vi "Describe Variant.vi"(11 "Variant":variant) -> (1 "Type Description":string, 2 "Description":string, 3 "Variant Description":string)   [LabVIEW 2020, in "LUnit Test Case.lvclass"]
uses:
  LUnit Test Case.lvclass
  <vilib>/Utility/Data Type/NI_Data Type.lvlib
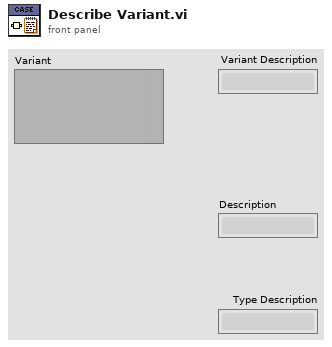
[diagram p1: front panel]
types:
  T1 = typedef "NI_Data Type.lvlib/Data Type.ctl" = enum8{"Invalid Type", "Void", "I8", "I16", "I32", "I64", "U8", "U16", "U32", "U64", "Single Float", "Double Float", "Extended Float", "Single Complex", "Double Complex", "Extended Complex", "Enum U8", "Enum U16", "Enum U32", "Enum U64", "Single Float With Unit", "Double Float With Unit", "Extended Float With Unit", "Single Complex with Unit", "Double Complex with Unit", "Extended Complex with Unit", "Boolean", "String", "Path", "Picture", "Tag", "Array", "Cluster", "Variant", "LV Variant", "Waveform", "Timestamp", "Digital Waveform", "Digital Data", "ExpressData", "Refnum", "External Data", "VI", "Poly VI", "LabVIEW Class Instance", "Fixed Point", "Set Collection", "Map Collection"}
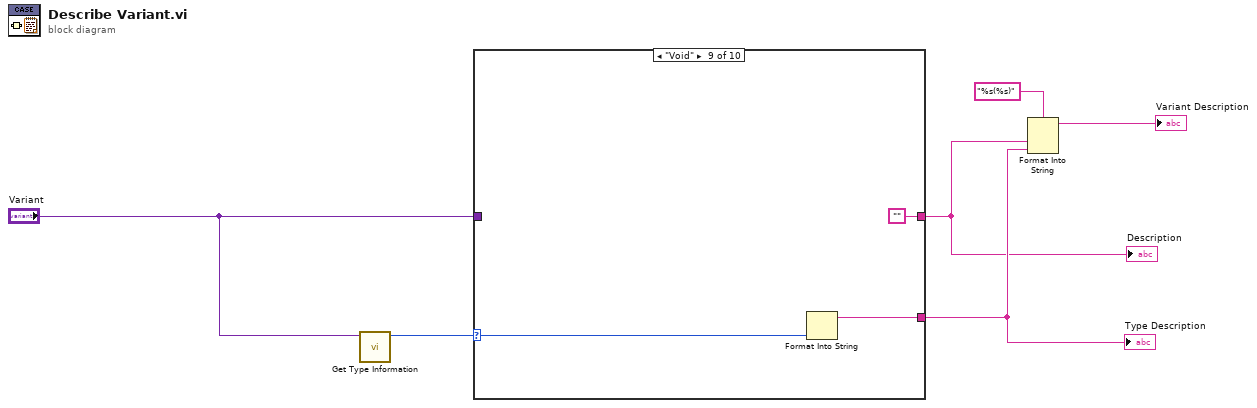
[diagram p0: block diagram]
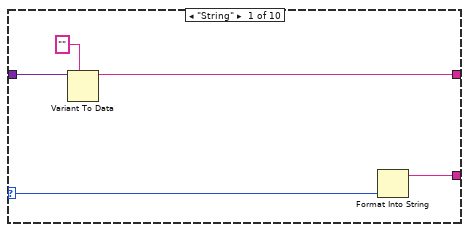
[diagram p2: hidden frame]
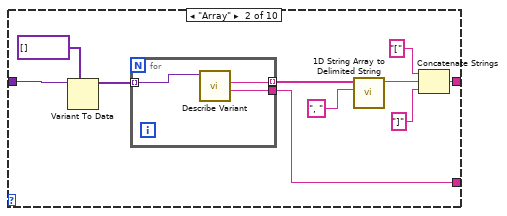
[diagram p3: hidden frame]
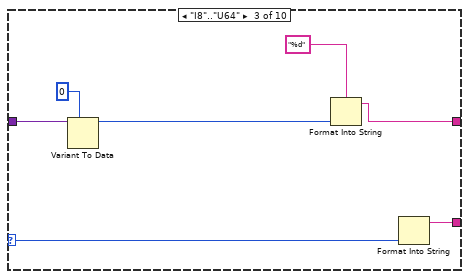
[diagram p4: hidden frame]
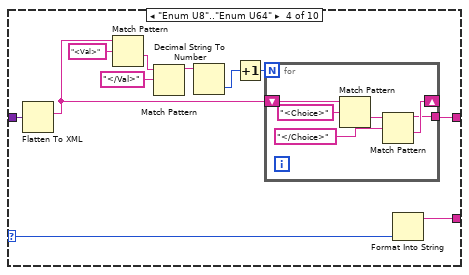
[diagram p5: hidden frame]
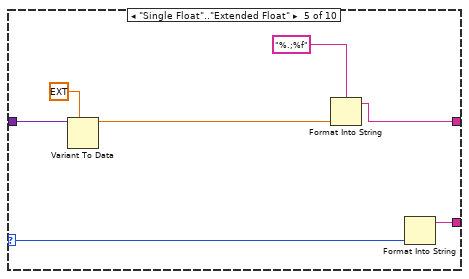
[diagram p6: hidden frame]
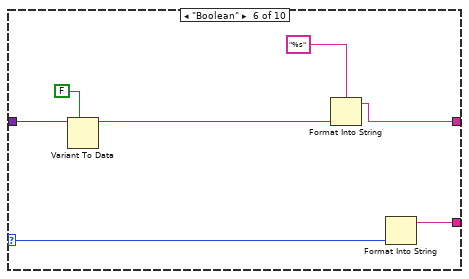
[diagram p7: hidden frame]
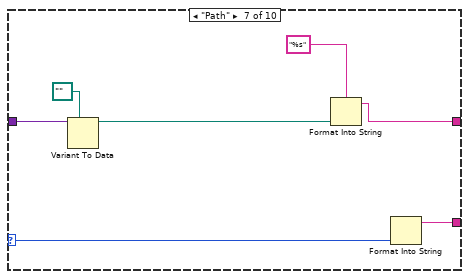
[diagram p8: hidden frame]
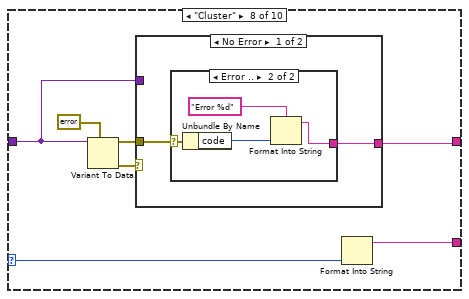
[diagram p9: hidden frame]
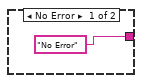
[diagram p10: hidden frame]
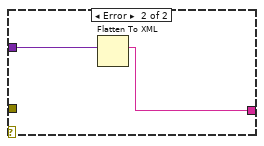
[diagram p11: hidden frame]
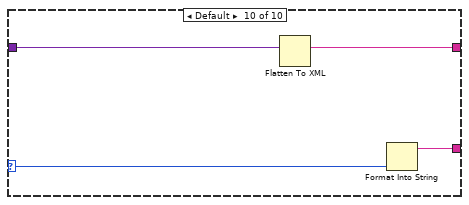
[diagram p12: hidden frame]
diagram:
  n1 = call <vilib>:"Get Type Information.vi"("variant"="Variant") -> ("type"=w5:T1)  [unwired: 6 in, 4 out]
  n2 = case shown="\"Void\"" w5 {
    selector: w5 -> [w7 _ w25 w41 w49 w56 w63 w74 w88 w89]
    tunnel: "Variant" -> [w11 w21 w31 w33 w55 w62 w69 w70 _ w92]
    tunnel: [w10 w15 w27 w32 w51 w58 w65 w72 "" w91] -> w2
    tunnel: [w8 w12 w26 w42 w50 w57 w64 w73 w87 w90] -> w4
    frame "String" {
      n3 = Variant To Data(type="", Variant=w11) -> (data=w10:string)  [unwired: 1 in, 1 out]
      n4 = Format Into String(w7) -> (resulting string=w8:string)  [unwired: 3 in, 1 out]
    }
    frame "Array" {
      n5 = Variant To Data(type=variant[] [], Variant=w21) -> (data=w19:variant[])  [unwired: 1 in, 1 out]
      n6 = for {
        tunnel: w19 -> [w24] mode=indexing
        tunnel: [w22] -> w17 mode=indexing
        tunnel: [w23] -> w12
        n7 = call "Describe Variant.vi"("Variant"=w24) -> ("Type Description"=w23:string, "Description"=w22:string)  [unwired: 8 in, 1 out]
      }
      n8 = call <vilib>:"1D String Array to Delimited String.vi"("delimiter"=", ", "string array"=w17) -> ("delimited string"=w16:string)  [unwired: 9 in]
      n9 = Concatenate Strings("[", w16, "]") -> (w15:string)
    }
    frame "I8".."U64" {
      n10 = Variant To Data(type=i64 0, Variant=w31) -> (data=w29:i64)  [unwired: 1 in, 1 out]
      n11 = Format Into String(format string="%d", w29) -> (resulting string=w27:string)  [unwired: 2 in, 1 out]
      n12 = Format Into String(w25) -> (resulting string=w26:string)  [unwired: 3 in, 1 out]
    }
    frame "Enum U8".."Enum U64" {
      n13 = Flatten To XML(6:w33) -> (2:w36:string)
      n14 = Match Pattern(string=w36, regular expression="<Val>" ("string")) -> (after substring=w37:string)  [unwired: 1 in, 3 out]
      n15 = Match Pattern(string=w37, regular expression="</Val>") -> (before substring=w38:string)  [unwired: 1 in, 3 out]
      n16 = Decimal String To Number(string=w38) -> (number=w39:i32)  [unwired: 2 in, 1 out]
      n17 = Increment(x=w39) -> (x+1=w40:i32)
      n18 = for {
        N: w40 -> [_]
        shift-right: [w44] -> _
        shift-left: w36 -> [w46]
        tunnel: [w43] -> w32
        n19 = Match Pattern(string=w46, regular expression="<Choice>" ("string")) -> (after substring=w48:string)  [unwired: 1 in, 3 out]
        n20 = Match Pattern(string=w48, regular expression="</Choice>") -> (before substring=w43:string, after substring=w44:string)  [unwired: 1 in, 2 out]
      }
      n21 = Format Into String(w41) -> (resulting string=w42:string)  [unwired: 3 in, 1 out]
    }
    frame "Single Float".."Extended Float" {
      n22 = Variant To Data(type=ext 0.0, Variant=w55) -> (data=w53:ext)  [unwired: 1 in, 1 out]
      n23 = Format Into String(format string="%.;%f", w53) -> (resulting string=w51:string)  [unwired: 2 in, 1 out]
      n24 = Format Into String(w49) -> (resulting string=w50:string)  [unwired: 3 in, 1 out]
    }
    frame "Boolean" {
      n25 = Variant To Data(type=FALSE, Variant=w62) -> (data=w60:bool)  [unwired: 1 in, 1 out]
      n26 = Format Into String(format string="%s", w60) -> (resulting string=w58:string)  [unwired: 2 in, 1 out]
      n27 = Format Into String(w56) -> (resulting string=w57:string)  [unwired: 3 in, 1 out]
    }
    frame "Path" {
      n28 = Variant To Data(type=path "", Variant=w69) -> (data=w67:path)  [unwired: 1 in, 1 out]
      n29 = Format Into String(format string="%s", w67) -> (resulting string=w65:string)  [unwired: 2 in, 1 out]
      n30 = Format Into String(w63) -> (resulting string=w64:string)  [unwired: 3 in, 1 out]
    }
    frame "Cluster" {
      n31 = Variant To Data(type=errorcluster {"status"=FALSE, "code"=0, "source"=""} ("error in"), Variant=w70) -> (data=w75:errorcluster, error out=w71:errorcluster)  [unwired: 1 in]
      n32 = case shown="No Error" w71 {
        tunnel: w75 -> [w78 _]
        tunnel: [w77 w84] -> w72
        tunnel: w70 -> [_ w85]
        frame No Error {
          n33 = case shown="Error .." w78 {
            selector: w78 -> [_ w83]
            tunnel: ["No Error" w81] -> w77
            frame No Error {
            }
            frame Error {
              n34 = Unbundle By Name(w83) -> ("code"=w82:i32)
              n35 = Format Into String(format string="Error %d", w82) -> (resulting string=w81:string)  [unwired: 2 in, 1 out]
            }
          }
        }
        frame Error {
          n36 = Flatten To XML(6:w85) -> (2:w84:string)
        }
      }
      n37 = Format Into String(w74) -> (resulting string=w73:string)  [unwired: 3 in, 1 out]
    }
    frame "Void" {
      n38 = Format Into String(w88) -> (resulting string=w87:string)  [unwired: 3 in, 1 out]
    }
    frame Default {
      n39 = Flatten To XML(6:w92) -> (2:w91:string)
      n40 = Format Into String(w89) -> (resulting string=w90:string)  [unwired: 3 in, 1 out]
    }
  }
  "Type Description" <- w4
  "Description" <- w2
  n41 = Format Into String(format string="%s(%s)", w2, w4) -> (resulting string=→"Variant Description":string)  [unwired: 2 in, 1 out]
